vi "LWXPS_PositionerAnalogTrackingVelocityParametersGet.vi"(0 "XPS Reference IN":refnum<k24>, 2 "Positioner Name":string, 5 "LabVIEW error IN":errorcluster) -> (8 "XPS Reference OUT":refnum<k24>, 10 "Returned error code":i32, 11 "LabVIEW error OUT":errorcluster, 12 "Analog Input Name":string, 13 "XPS Error String":string, 14 "Offset":dbl, 15 "Scale":dbl, 16 "Dead Band Threshold":dbl, 17 "Order":i32, 18 "Velocity":dbl, 19 "Acceleration":dbl)   [LabVIEW 2014]
uses:
  D:/XPSQ8_LabView_Library/Development/Source/Dll/Newport.XPS.CommandInterface.dll
  Dll/Newport.XPS.CommandInterface.dll
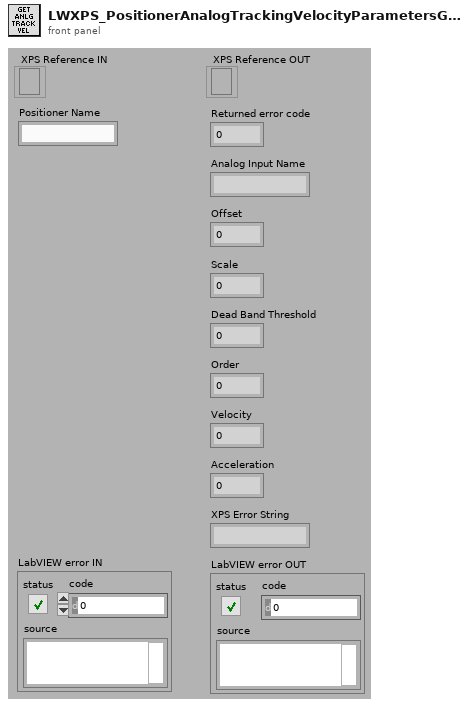
[diagram p1: front panel]
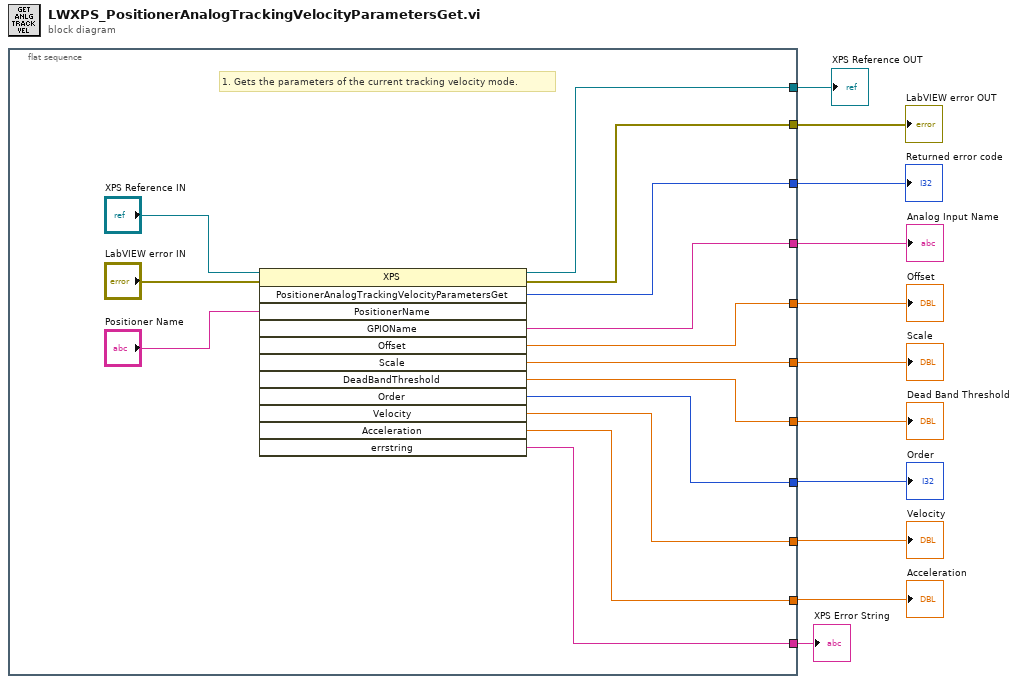
[diagram p0: block diagram]
diagram:
  n1 = flat-sequence {
    tunnel: [w20] -> w8
    tunnel: [w12] -> w11
    tunnel: [w24] -> w10
    tunnel: [w23] -> w9
    tunnel: [w19] -> w7
    tunnel: [w18] -> w6
    tunnel: [w17] -> w5
    tunnel: [w16] -> w4
    tunnel: [w15] -> w3
    tunnel: [w13] -> w2
    tunnel: [w14] -> w1
    frame #0 {
      # "1. Gets the parameters of the current tracking velocity mode."
      n2 = invoke class="XPS" method="PositionerAnalogTrackingVelocityParametersGet"(reference="XPS Reference IN", error in="LabVIEW error IN", "PositionerName"="Positioner Name") -> (reference out=w12:refnum<k24>, error out=w24:errorcluster, "PositionerAnalogTrackingVelocityParametersGet"=w23:i32, "GPIOName"=w20:string, "Offset"=w19:dbl, "Scale"=w18:dbl, "DeadBandThreshold"=w17:dbl, "Order"=w16:i32, "Velocity"=w15:dbl, "Acceleration"=w13:dbl, "errstring"=w14:string)  [unwired: 9 in, 1 out]
    }
  }
  "XPS Error String" <- w1
  "XPS Reference OUT" <- w11
  "LabVIEW error OUT" <- w10
  "Returned error code" <- w9
  "Analog Input Name" <- w8
  "Offset" <- w7
  "Scale" <- w6
  "Velocity" <- w3
  "Acceleration" <- w2
  "Dead Band Threshold" <- w5
  "Order" <- w4
